vi "F-Truncat-ILPF.vi"() -> ()   [LabVIEW 2014]
doc: "Use this template to build a VI to use as a subVI."
uses:
  <vilib>/vision/NI_Vision_Development_Module.lvlib
panel:
  out "|F(u,v)H(u,v)|":T1(plugin-control)
  out "g(x,y)":T1(plugin-control)
  out "IF(u,v)I":T1(plugin-control)
  out "f(x,y)":T1(plugin-control)
  # ":: MVi Framework V1.0 ::\nAuthor:Gaoke Yang\nEmail: gaoke.yang@yahoo.com\nWeb: www.mvicontrol.com\nCopyright (C) 2015, MVI Technologies All Rights Reserved"
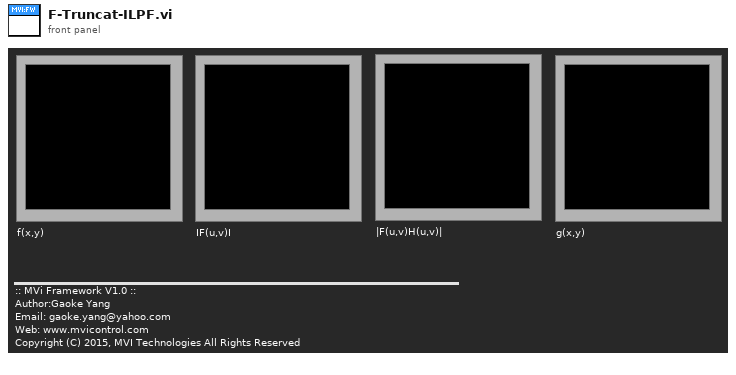
[diagram p1: front panel]
types:
  T1 = typedef "IMAQ Image.ctl" = refnum<image>
  T2 = typedef "Image Type" = u32
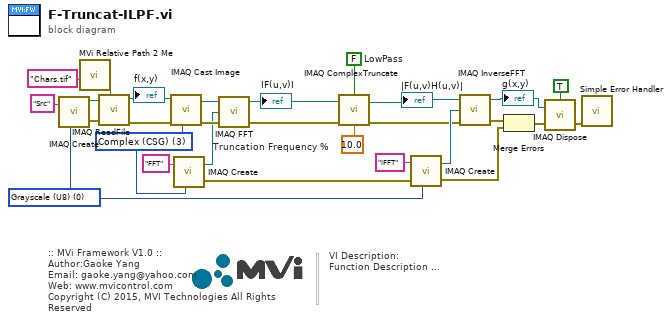
[diagram p0: block diagram]
diagram:
  w7 = sgl 10.0  # Truncation Frequency %
  w8 = FALSE  # LowPass
  w1 = T2 0 items=["Grayscale (U8)", "Grayscale (I16)", "Grayscale (SGL)", "Complex (CSG)", "RGB (U32)", "HSL (U32)", "RGB (U64)", "Grayscale (U16)"] ("Image Type")
  w9 = T2 3 items=["Grayscale (U8)", "Grayscale (I16)", "Grayscale (SGL)", "Complex (CSG)", "RGB (U32)", "HSL (U32)", "RGB (U64)", "Grayscale (U16)"] ("Image Type")
  # "VI Description:\nFunction Description ..."
  # ":: MVi Framework V1.0 ::\nAuthor:Gaoke Yang\nEmail: gaoke.yang@yahoo.com\nWeb: www.mvicontrol.com\nCopyright (C) 2015, MVI Technologies All Rights Reserved"
  n1 = call "IMAQ Create"("Image Name"="Src" ("name or relative path"), "Image Type"=w1) -> ("New Image"=w25:T1, "error out"=w24:errorcluster)  [unwired: 2 in, 1 out]
  n2 = call "MVi Relative Path 2 Me.vi"("Relative Path"="Chars.tif" ("name or relative path")) -> ("Appended Dir"=w21:path)  [unwired: 5 in, 1 out]
  n3 = call "IMAQ ReadFile"("File Path"=w21, "error in (no error)"=w24, "Image"=w25) -> ("error out"=w18:errorcluster, "Image Out"=w17:T1)  [unwired: 4 in, 3 out]
  "f(x,y)" <- w17
  n4 = call "IMAQ Cast Image"("Image Type"=w9, "error in (no error)"=w18, "Image Src"=w17) -> ("error out"=w20:errorcluster, "Image Dst Out"=w16:T1)  [unwired: 7 in]
  n5 = call "IMAQ Create"("Image Name"="FFT" ("name or relative path"), "Image Type"=w9) -> ("New Image"=w15:T1, "error out"=w4:errorcluster)  [unwired: 2 in, 1 out]
  n6 = call "IMAQ FFT"("error in (no error)"=w20, "Image Dst"=w15, "Image Src"=w16) -> ("error out"=w6:errorcluster, "Image Dst Out"=w5:T1)  [unwired: 1 in]
  "IF(u,v)I" <- w5
  n7 = call "IMAQ ComplexTruncate"("error in (no error)"=w6, "Truncation Frequency %"=w7, "Image Src"=w5, "Low pass/High pass (Low pass)"=w8) -> ("error out"=w3:errorcluster, "Image Dst Out"=w2:T1)  [unwired: 3 in]
  "|F(u,v)H(u,v)|" <- w2
  n8 = call "IMAQ Create"("Image Name"="iFFT" ("name or relative path"), "Image Type"=w1, "error in (no error)"=w4) -> ("New Image"=w13:T1, "error out"=w10:errorcluster)  [unwired: 1 in, 1 out]
  n9 = call "IMAQ InverseFFT"("error in (no error)"=w3, "Image Dst"=w13, "Image Src"=w2) -> ("error out"=w12:errorcluster, "Image Dst Out"=w11:T1)  [unwired: 1 in]
  "g(x,y)" <- w11
  n10 = Merge Errors(w12, w10) -> (w19:errorcluster)
  n11 = call "IMAQ Dispose"("All Images? (No)"=TRUE, "Image"=w11, "error in (no error)"=w19) -> ("error out"=w26:errorcluster)  [unwired: 3 out]
  n12 = call <vilib>:"Simple Error Handler.vi"("error in (no error)"=w26) -> ()  [unwired: 1 in, 8 out]
